vi "VIE.Module.Queued Message Handler.dqClass_TestClassPerformance(Locked).vi"() -> ()   [LabVIEW 2010, in "VIE.Module.Queued Message Handler.QueuedMessageHandler.dqGOOPClass.lvlib"]
doc: "This tests class performance for generating, creating, obtaining, setting and deleting n class objects."
uses:
  VIE.Module.Queued Message Handler.QueuedMessageHandler.dqGOOPClass.lvlib
  VIE.Module.Queued Message Handler.dqClass_ObjectData.ctl
panel:
  in  "error in (no error)":errorcluster
  out "total":u32
  out "Delete Pass":bool
  out "Get Data Modify Pass":bool
  out "Get Data Pass":bool
  out "error out":errorcluster
  in  "Number":i32=1000
  out "delete":u32
  out "set (Locked)":u32
  out "get (Locked)":u32
  out "create":u32
  out "generate data":u32
  in  "data":T1
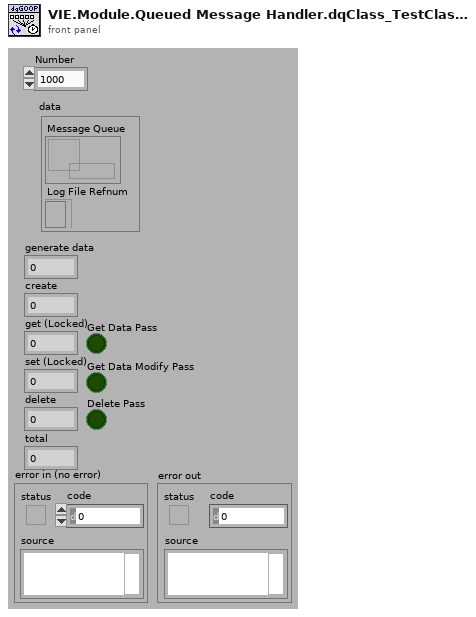
[diagram p1: front panel]
types:
  T1 = typedef "VIE.Module.Queued Message Handler.QueuedMessageHandler.dqGOOPClass.lvlib/VIE.Module.Queued Message Handler.dqClass_ObjectData.ctl" = cluster{"Message Queue":refnum<queue>, "Log File Refnum":refnum<file>}
  T2 = typedef "VIE.Module.Queued Message Handler.QueuedMessageHandler.dqGOOPClass.lvlib/VIE.Module.Queued Message Handler.dqClass_ObjectReference.ctl" = refnum<k1>
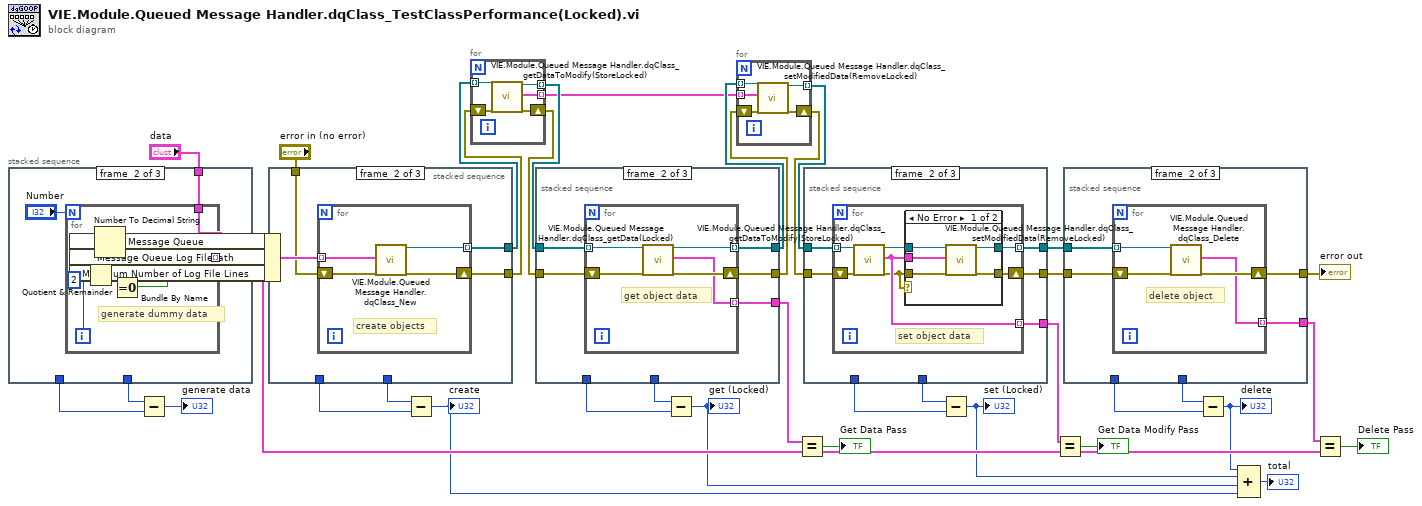
[diagram p0: block diagram]
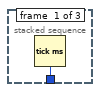
[diagram p2: hidden frame]
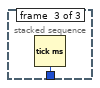
[diagram p3: hidden frame]
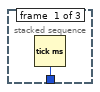
[diagram p4: hidden frame]
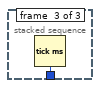
[diagram p6: hidden frame]
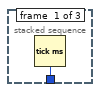
[diagram p7: hidden frame]
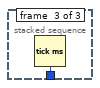
[diagram p8: hidden frame]
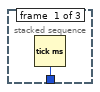
[diagram p9: hidden frame]
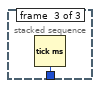
[diagram p10: hidden frame]
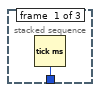
[diagram p11: hidden frame]
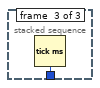
[diagram p12: hidden frame]
diagram:
  n1 = stacked-sequence {
    tunnel: [w38 _ _] -> w34
    tunnel: [_ _ w49] -> w35
    tunnel: [_ w40 _] -> w17
    tunnel: "data" -> [_ w41 _]
    frame #0 {
      n2 = Tick Count (ms)() -> (millisecond timer value=w38:u32)
    }
    frame #1 {
      n3 = for {
        N: "Number" -> [_]
        tunnel: w41 -> [w48]
        tunnel: [w47] -> w40 mode=indexing
        i -> [w45]
        # "generate dummy data"
        n4 = Quotient & Remainder(x=w45, y=2) -> (x-y*floor(x/y)=w43:i32)  [unwired: 1 out]
        n5 = Number To Decimal String(number=w45) -> (decimal integer string=w46:string)  [unwired: 1 in]
        n6 = Equal To 0?(x=w43) -> (x = 0?=w42:bool)
        n7 = Bundle By Name(cluster=w48, "Message Queue"=w46, "Message Queue Log FilePath"=w45, "Maximum Number of Log File Lines"=w42) -> (w47:T1)
      }
    }
    frame #2 {
      n8 = Tick Count (ms)() -> (millisecond timer value=w49:u32)
    }
  }
  n9 = Subtract(x=w35, y=w34) -> (x-y=→"generate data":u32)
  n10 = stacked-sequence {
    tunnel: [w50 _ _] -> w37
    tunnel: [_ _ w59] -> w36
    tunnel: w17 -> [_ w54 _]
    tunnel: [_ w53 _] -> w6
    tunnel: [_ w52 _] -> w9
    tunnel: "error in (no error)" -> [_ w51 _]
    frame #0 {
      n11 = Tick Count (ms)() -> (millisecond timer value=w50:u32)
    }
    frame #1 {
      n12 = for {
        shift-right: [w57] -> w53
        shift-left: w51 -> [w58]
        tunnel: w54 -> [w56] mode=indexing
        tunnel: [w55] -> w52 mode=indexing
        # "create objects"
        n13 = call "VIE.Module.Queued Message Handler.dqClass_New.vi"("data"=w56, "error in (no error)"=w58) -> ("reference"=w55:T2, "error out"=w57:errorcluster)  [unwired: 16 in]
      }
    }
    frame #2 {
      n14 = Tick Count (ms)() -> (millisecond timer value=w59:u32)
    }
  }
  n15 = Subtract(x=w36, y=w37) -> (x-y=w12:u32)
  "create" <- w12
  n16 = for {
    shift-right: [w63] -> w7
    shift-left: w6 -> [w64]
    tunnel: w9 -> [w62] mode=indexing
    tunnel: [w61] -> w8 mode=indexing
    tunnel: [w60] -> w1 mode=indexing
    n17 = call "VIE.Module.Queued Message Handler.dqClass_getDataToModify(StoreLocked).vi"("reference"=w62, "error in (no error)"=w64) -> ("duplicate reference"=w61:T2, "data"=w60:T1, "error out"=w63:errorcluster)  [unwired: 14 in, 1 out]
  }
  n18 = stacked-sequence {
    tunnel: [w65 _ _] -> w33
    tunnel: [_ _ w76] -> w32
    tunnel: w7 -> [_ w70 _]
    tunnel: [_ w69 _] -> w5
    tunnel: w8 -> [_ w68 _]
    tunnel: [_ w67 _] -> w4
    tunnel: [_ w66 _] -> w22
    frame #0 {
      n19 = Tick Count (ms)() -> (millisecond timer value=w65:u32)
    }
    frame #1 {
      n20 = for {
        shift-right: [w74] -> w69
        shift-left: w70 -> [w75]
        tunnel: w68 -> [w73] mode=indexing
        tunnel: [w72] -> w67 mode=indexing
        tunnel: [w71] -> w66 mode=indexing
        # "get object data"
        n21 = call "VIE.Module.Queued Message Handler.dqClass_getData(Locked).vi"("reference"=w73, "error in (no error)"=w75) -> ("duplicate reference"=w72:T2, "data"=w71:T1, "error out"=w74:errorcluster)  [unwired: 13 in, 2 out]
      }
    }
    frame #2 {
      n22 = Tick Count (ms)() -> (millisecond timer value=w76:u32)
    }
  }
  n23 = Subtract(x=w32, y=w33) -> (x-y=w13:u32)
  "get (Locked)" <- w13
  n24 = for {
    shift-right: [w80] -> w2
    shift-left: w5 -> [w81]
    tunnel: w4 -> [w79] mode=indexing
    tunnel: [w78] -> w3 mode=indexing
    tunnel: w1 -> [w77] mode=indexing
    n25 = call "VIE.Module.Queued Message Handler.dqClass_setModifiedData(RemoveLocked).vi"("reference"=w79, "data"=w77, "error in (no error)"=w81) -> ("duplicate reference"=w78:T2, "error out"=w80:errorcluster)  [unwired: 15 in]
  }
  n26 = Equal?(x=w22, y=w17) -> (x = y?=→"Get Data Pass":bool)
  n27 = stacked-sequence {
    tunnel: [w82 _ _] -> w31
    tunnel: [_ _ w102] -> w30
    tunnel: w2 -> [_ w87 _]
    tunnel: [_ w86 _] -> w27
    tunnel: w3 -> [_ w85 _]
    tunnel: [_ w84 _] -> w26
    tunnel: [_ w83 _] -> w18
    frame #0 {
      n28 = Tick Count (ms)() -> (millisecond timer value=w82:u32)
    }
    frame #1 {
      n29 = for {
        shift-right: [w94] -> w86
        shift-left: w87 -> [w90]
        tunnel: w85 -> [w92] mode=indexing
        tunnel: [w93] -> w84 mode=indexing
        tunnel: [w89] -> w83 mode=indexing
        # "set object data"
        n30 = call "VIE.Module.Queued Message Handler.dqClass_getDataToModify(StoreLocked).vi"("reference"=w92, "error in (no error)"=w90) -> ("duplicate reference"=w91:T2, "data"=w89:T1, "error out"=w88:errorcluster)  [unwired: 14 in, 1 out]
        n31 = case shown="No Error" w88 {
          tunnel: [w99 w100] -> w94
          tunnel: [w98 w101] -> w93
          tunnel: w91 -> [w97 w101]
          tunnel: w89 -> [w96 _]
          tunnel: w88 -> [w95 w100]
          frame No Error {
            n32 = call "VIE.Module.Queued Message Handler.dqClass_setModifiedData(RemoveLocked).vi"("reference"=w97, "data"=w96, "error in (no error)"=w95) -> ("duplicate reference"=w98:T2, "error out"=w99:errorcluster)  [unwired: 15 in]
          }
          frame Error {
          }
        }
      }
    }
    frame #2 {
      n33 = Tick Count (ms)() -> (millisecond timer value=w102:u32)
    }
  }
  n34 = Subtract(x=w30, y=w31) -> (x-y=w14:u32)
  "set (Locked)" <- w14
  n35 = Equal?(x=w18, y=w17) -> (x = y?=→"Get Data Modify Pass":bool)
  n36 = stacked-sequence {
    tunnel: [w103 _ _] -> w29
    tunnel: [_ _ w112] -> w28
    tunnel: w27 -> [_ w107 _]
    tunnel: w26 -> [_ w106 _]
    tunnel: [_ w105 _] -> w23
    tunnel: [_ w104 _] -> w16
    frame #0 {
      n37 = Tick Count (ms)() -> (millisecond timer value=w103:u32)
    }
    frame #1 {
      n38 = for {
        shift-right: [w110] -> w105
        shift-left: w107 -> [w111]
        tunnel: w106 -> [w109] mode=indexing
        tunnel: [w108] -> w104 mode=indexing
        # "delete object"
        n39 = call "VIE.Module.Queued Message Handler.dqClass_Delete.vi"("reference"=w109, "error in (no error)"=w111) -> ("data"=w108:T1, "error out"=w110:errorcluster)  [unwired: 15 in, 1 out]
      }
    }
    frame #2 {
      n40 = Tick Count (ms)() -> (millisecond timer value=w112:u32)
    }
  }
  "error out" <- w23
  n41 = Subtract(x=w28, y=w29) -> (x-y=w15:u32)
  "delete" <- w15
  n42 = Compound Arithmetic op=ADD(w15, w14, w13, w12) -> (→"total":u32)
  n43 = Equal?(x=w16, y=w17) -> (x = y?=→"Delete Pass":bool)
